vi "ATF-Storage URL NS.vi"(7 "Enum":enum16{"Init", "Read", "Write"}(ring)=enum."Read", 8 "error IN":errorcluster, 11 "writer endpoint":refnum<k21>) -> (0 "error OUT":errorcluster, 3 "writer endpoint R":refnum<k21>)   [LabVIEW 2022 SP3]
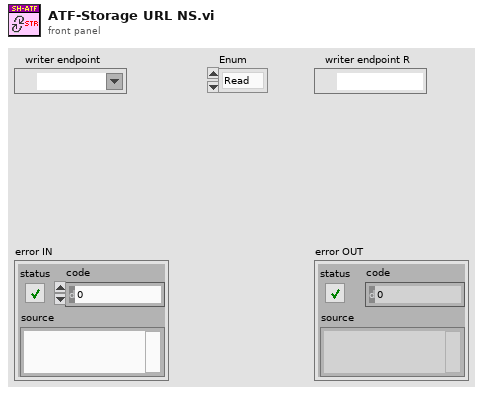
[diagram p1: front panel]
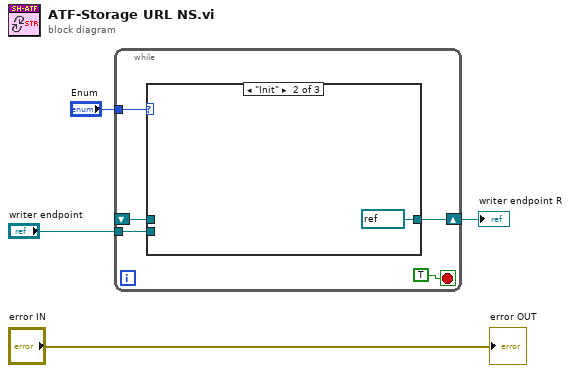
[diagram p0: block diagram]
diagram:
  n1 = while {
    tunnel: "Enum" -> [w8]
    shift-right: [w6] -> w2
    shift-left: _ -> [w7]
    tunnel: "writer endpoint" -> [w5]
    stop <- TRUE stop-if-true
    n2 = case shown="\"Init\"" w8 {
      tunnel: w7 -> [w10 _ _]
      tunnel: [w10 refnum<k21> refnum ("writer endpoint") w12] -> w6
      tunnel: w5 -> [_ _ w12]
      frame "Read", Default {
      }
      frame "Init" {
      }
      frame "Write" {
      }
    }
  }
  "writer endpoint R" <- w2
  "error OUT" <- "error IN"
